vi "UnboxI32Array.vi"(8 "error in (no error)":errorcluster, 9 "Items":refnum<class>[](array[class])) -> (0 "error out":errorcluster, 1 "Array":i32[](array[numeric]))   [LabVIEW 2013, in "ListImp_Populated.lvclass"]
uses:
  ListImp_Populated.lvclass
  source/LapDog.Collections.Common/I32/I32.lvclass
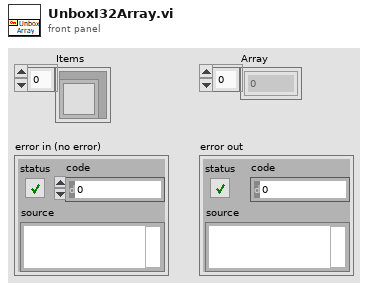
[diagram p1: front panel]
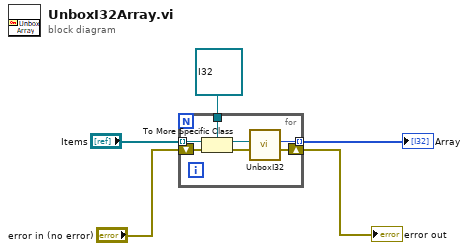
[diagram p0: block diagram]
diagram:
  n1 = for {
    tunnel: "Items" -> [w10] mode=indexing
    tunnel: [w6] -> w4 mode=indexing
    shift-right: [w9] -> w5
    shift-left: "error in (no error)" -> [w11]
    tunnel: refnum<class "I32.lvclass"> refnum ("LapDog.Collections.v_.Common.lvlib:I32.lvclass") -> [w8]
    n2 = To More Specific Class(target class=w8, reference=w10, error in=w11) -> (specific class reference=w7:refnum<class "I32.lvclass">, error out=w9:errorcluster)
    n3 = call "UnboxI32.vi"("I32 in"=w7) -> ("Numeric"=w6:i32)  [unwired: 10 in]
  }
  "error out" <- w5
  "Array" <- w4
